vi "SCC Compare VIs.vi"(4 "version":string, 6 "interactive? (F)":bool, 7 "application reference":refnum<vi>, 8 "error in (no error)":errorcluster, 9 "compare options":T1={"VI Attributes"=FALSE, "Front Panel"=TRUE, "FP position/size"=FALSE, "Block Diagram"=TRUE, "BD cosmetic"=FALSE, "BD position/size"=FALSE}, 10 "VI path":path, 11 "source control reference in":T2) -> (0 "error out":errorcluster, 2 "status message":string, 3 "source control reference out":T2, 5 "file differs?":bool)   [LabVIEW 2017, in "NI_SCC.lvlib"]
doc: "Returns the difference between the specified VI and by default, the latest version of the VI in source control."
uses:
  <vilib>/SourceControl/sccapi/NI_SCC.lvlib
  <vilib>/SourceControl/sccapi/SCCAPI Refnum.ctl
  <vilib>/SourceControl/sccapi/SCCAPI VI Compare Options.ctl
  <vilib>/SourceControl/sccapi/SCCAPI SCC Provider Functionality.ctl
  <vilib>/SourceControl/support/SCCSup Message Strings GLBL.vi
  <vilib>/Utility/lvfile.llb/NI_FileType.lvlib
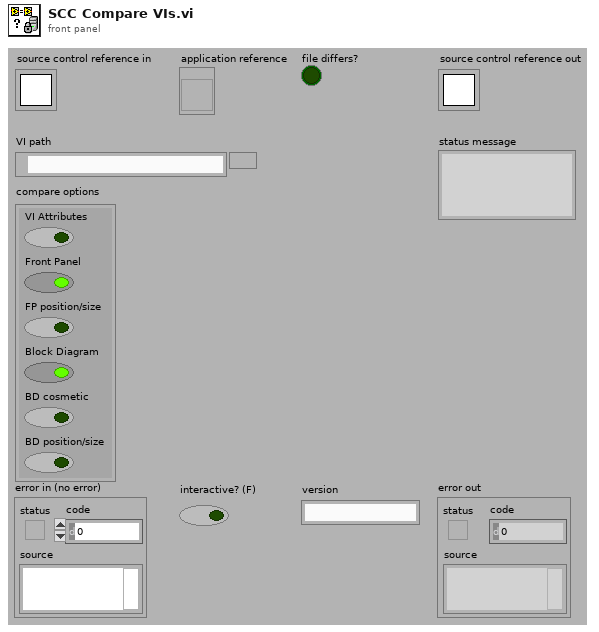
[diagram p1: front panel]
types:
  T1 = typedef "NI_SCC.lvlib/SCCAPI VI Compare Options.ctl" = cluster{"VI Attributes":bool, "Front Panel":bool, "FP position/size":bool, "Block Diagram":bool, "BD cosmetic":bool, "BD position/size":bool}
  T2 = typedef "NI_SCC.lvlib/SCCAPI Refnum.ctl" = refnum<k1>
  T3 = typedef "NI_SCC.lvlib/SCCAPI SCC Provider Functionality.ctl" = enum16{"Advanced - Get Latest", "Advanced - CheckOut", "Advanced - CheckIn", "Advanced - UndoCheckOut", "Advanced - Add", "Advanced - Remove", "Advanced - FileCompare", "Advanced - FileHistory", "Advanced - FileProperties", "Advanced - ConfigOptions", "Run SCC", "Configure Project", "Comment on CheckOut", "Comment on CheckIn", "Comment on Add", "Comment on Remove", "Keep Checked Out", "Get File Copy", "Multifile History"}
  T4 = typedef "NI_SCC.lvlib/SCCAPI SCC File Status.ctl" = cluster{"in source control?":bool, "checked out by user?":bool, "checked out by other?":bool, "out of date?":bool, "deleted?":bool}
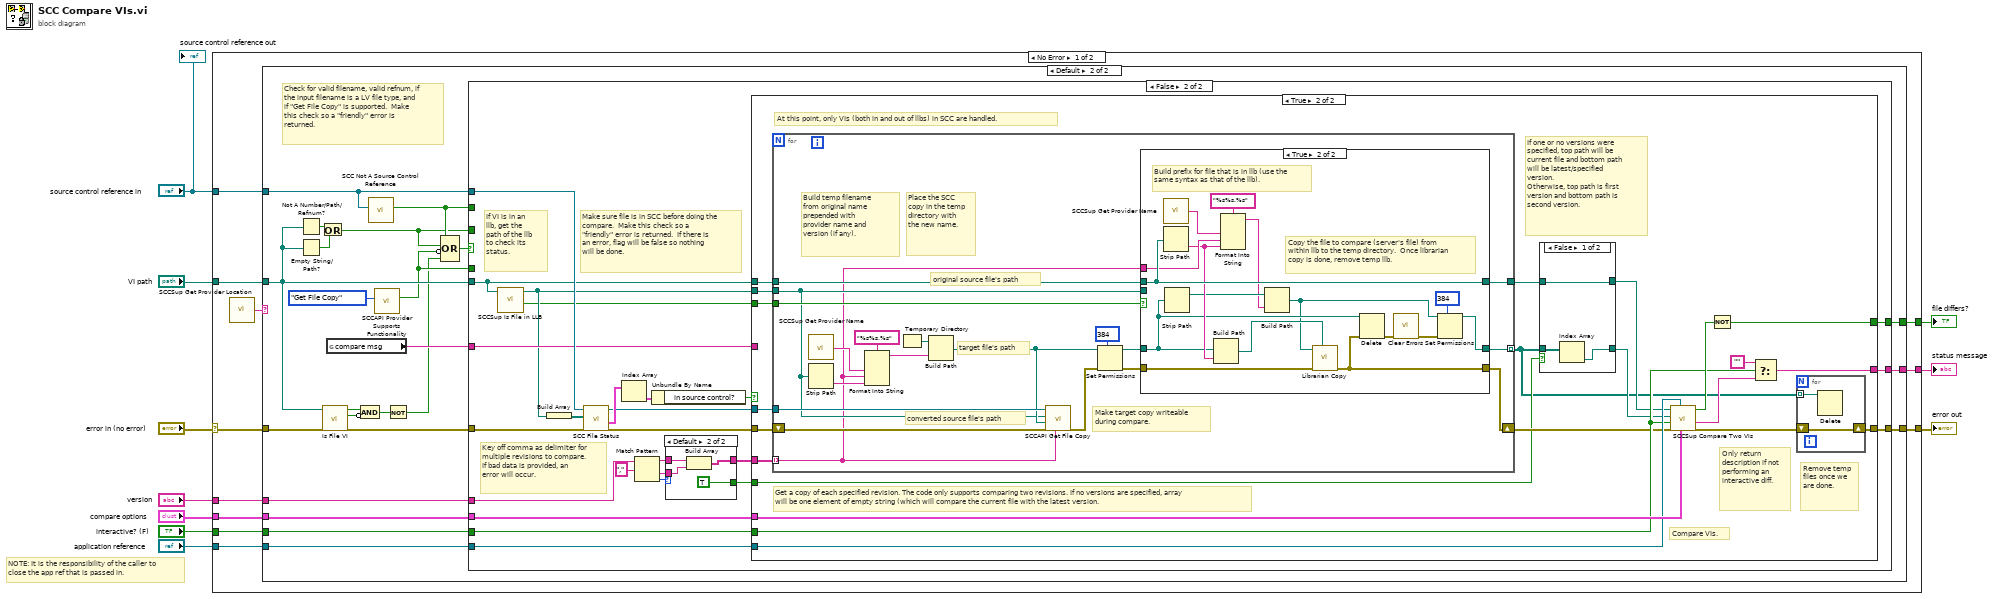
[diagram p0: block diagram]
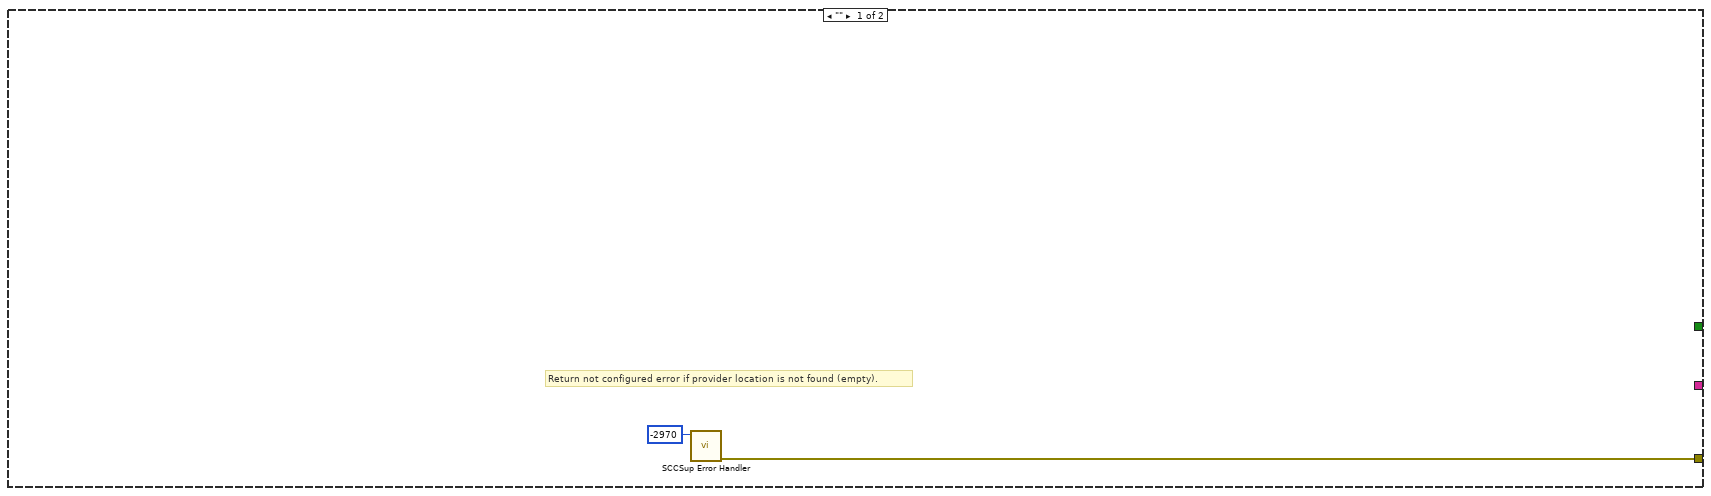
[diagram p2: hidden frame]
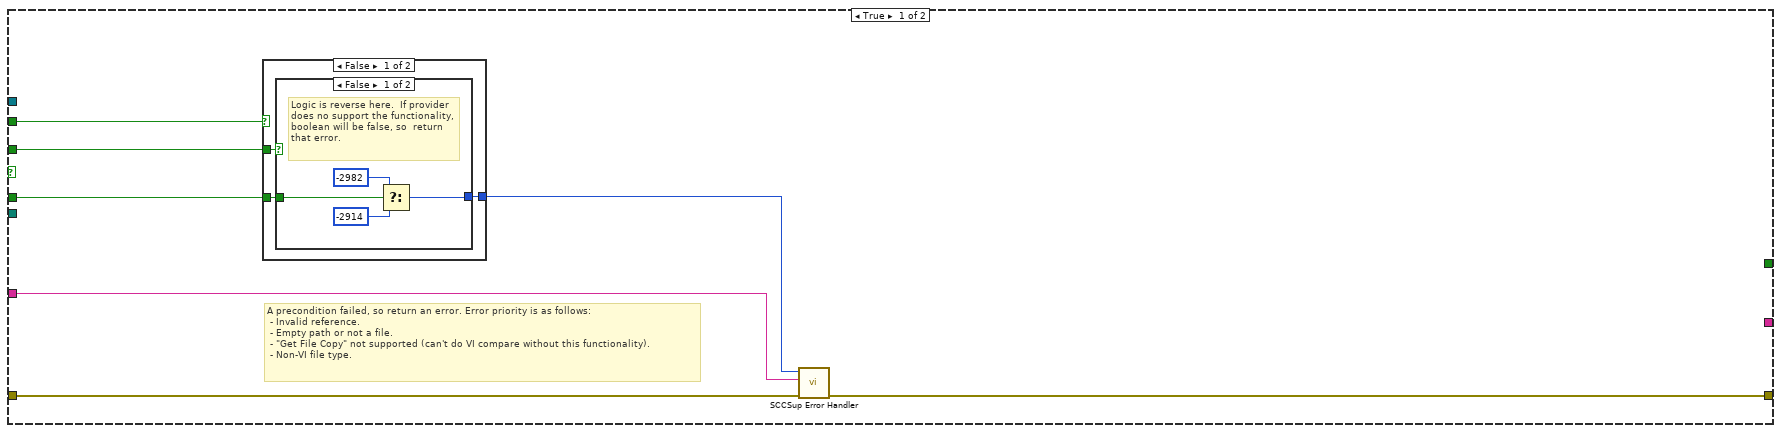
[diagram p3: hidden frame]
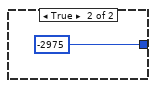
[diagram p4: hidden frame]
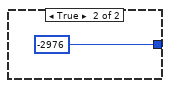
[diagram p5: hidden frame]
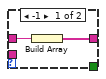
[diagram p6: hidden frame]
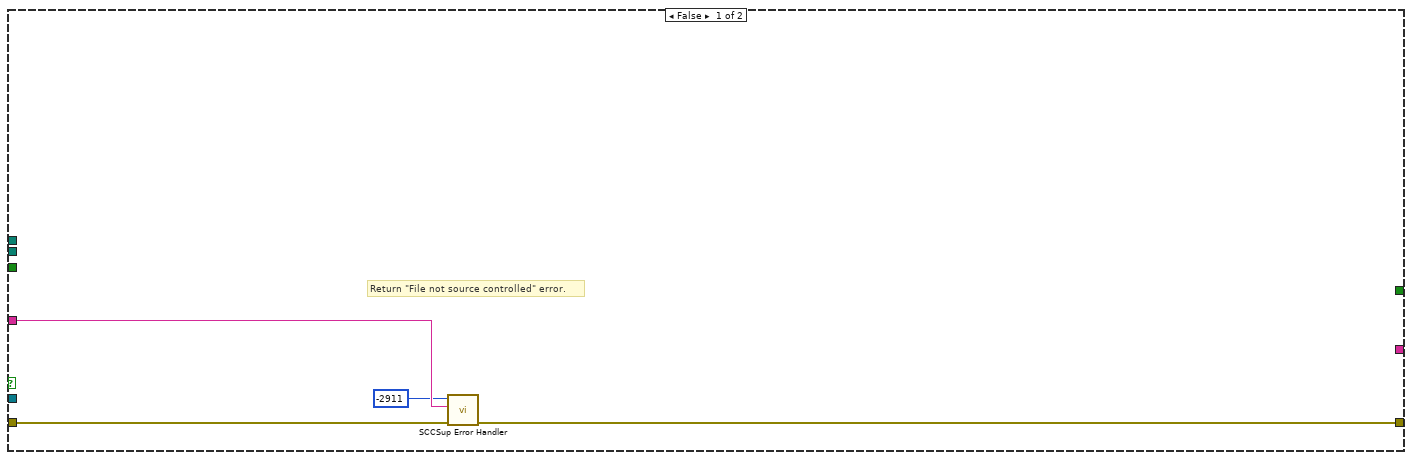
[diagram p7: hidden frame]
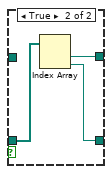
[diagram p8: hidden frame]
diagram:
  # "NOTE: It is the responsibility of the caller to close the app ref that is passed in."
  n1 = case shown="No Error" "error in (no error)" {
    selector: "error in (no error)" -> [w14 w166]
    tunnel: [w18 w166] -> w4
    tunnel: "source control reference in" -> [w21 _]
    tunnel: [w20 _] -> w3
    tunnel: "VI path" -> [w13 _]
    tunnel: [w19 _] -> w2
    tunnel: "compare options" -> [w16 _]
    tunnel: "interactive? (F)" -> [w17 _]
    tunnel: "version" -> [w15 _]
    tunnel: "application reference" -> [w12 _]
    frame No Error {
      n2 = call <vilib>:"SCCSup Get Provider Location.vi"() -> ("provider location"=w11:string)  [unwired: 6 in]
      n3 = case shown="Default" w11 {
        tunnel: w21 -> [_ w44]
        tunnel: [_ w41] -> w20
        tunnel: [_ w40] -> w19
        tunnel: [w22 w39] -> w18
        tunnel: w17 -> [_ w38]
        tunnel: w16 -> [_ w37]
        tunnel: w15 -> [_ w36]
        tunnel: w14 -> [_ w34]
        tunnel: w13 -> [_ w32]
        tunnel: w12 -> [_ w28]
        frame "" {
          # "Return not configured error if provider location is not found (empty)."
          n4 = call <vilib>:"SCCSup Error Handler.vi"("scc error code"=-2970 ("code")) -> ("error out"=w22:errorcluster)  [unwired: 10 in]
        }
        frame Default {
          # "Check for valid filename, valid refnum, if the input filename is a LV file type, and if \"Get File Copy\" is supported.  Make this check so a \"friendly\" error is returned."
          n5 = Not A Number/Path/Refnum?(number/path/refnum=w32) -> (NaN/Path/Refnum?=w46:bool)
          n6 = Empty String/Path?(string/path=w32) -> (empty?=w45:bool)
          n7 = Or(x=w46, y=w45) -> (x .or. y?=w31:bool)
          n8 = call <vilib>:"Is File VI.vi"("error in (no error)"=w34, "path"=w32) -> ("error out"=w33:errorcluster, "Is Class Private Data Control?"=w25:bool, "Is VI?"=w26:bool)  [unwired: 7 in]
          n9 = global read "SCCSup Message Strings GLBL.vi" "compare msg"() -> (w35:string)
          n10 = Compound Arithmetic op=AND(w26, invert w25) -> (w24:bool)
          n11 = call <vilib>:"SCC Not A Source Control Reference.vi"("source control reference in"=w44) -> ("not a source control reference?"=w42:bool)  [unwired: 9 in, 1 out]
          n12 = call <vilib>:"SCCAPI Provider Supports Functionality.vi"("functionality"=SCCAPI_SCC_Provider_Functionality."Get File Copy") -> ("provider supports?"=w29:bool)  [unwired: 9 in, 1 out]
          n13 = Not(x=w24) -> (.not. x?=w27:bool)
          n14 = Compound Arithmetic op=OR(w42, w31, invert w29, w27) -> (w43:bool)
          n15 = case shown="False" w43 {
            tunnel: w44 -> [_ w79]
            tunnel: [_ w80] -> w41
            tunnel: w32 -> [_ w72]
            tunnel: w42 -> [w50 _]
            tunnel: [_ w81] -> w40
            tunnel: w33 -> [w53 w76]
            tunnel: [w52 w82] -> w39
            tunnel: w38 -> [_ w87]
            tunnel: w37 -> [_ w86]
            tunnel: w36 -> [_ w68]
            tunnel: w35 -> [w51 w77]
            tunnel: w31 -> [w49 _]
            tunnel: w29 -> [w47 _]
            tunnel: w28 -> [_ w73]
            frame True {
              # "A precondition failed, so return an error. Error priority is as follows:\n - Invalid reference.  \n - Empty path or not a file.\n - \"Get File Copy\" not supported (can't do VI compare without this functionality).\n - Non-VI file type."
              n16 = case shown="False" w50 {
                tunnel: w49 -> [w54 _]
                tunnel: [w56 -2976 ("result")] -> w48
                tunnel: w47 -> [w55 _]
                frame False {
                  n17 = case shown="False" w54 {
                    tunnel: [w58 -2975 ("result")] -> w56
                    tunnel: w55 -> [w57 _]
                    frame False {
                      # "Logic is reverse here.  If provider does no support the functionality, boolean will be false, so  return that error."
                      n18 = Select(t=-2982 ("result"), s=w57, f=-2914 ("result")) -> (s? t:f=w58:i32)
                    }
                    frame True {
                    }
                  }
                }
                frame True {
                }
              }
              n19 = call <vilib>:"SCCSup Error Handler.vi"("error in (no error)"=w53, "operation message"=w51, "scc error code"=w48) -> ("error out"=w52:errorcluster)  [unwired: 8 in]
            }
            frame False {
              # "Key off comma as delimiter for multiple revisions to compare. If bad data is provided, an error will occur."
              # "If VI is in an llb, get the path of the llb to check its status."
              # "Make sure file is in SCC before doing the compare.  Make this check so a \"friendly\" error is returned.  If there is an error, flag will be false so nothing will be done."
              n20 = call <vilib>:"SCCSup Is File in LLB.vi"("Path"=w72) -> ("is in LLB?"=w70:bool, "converted path"=w71:path)  [unwired: 9 in]
              n21 = Build Array(w71) -> (w85:path[])
              n22 = call <vilib>:"SCC File Status.vi"("error in (no error)"=w76, "files"=w85, "source control reference in"=w79) -> ("error out"=w74:errorcluster, "file status"=w83:T4[], "source control reference out"=w78:T2)  [unwired: 4 in, 2 out]
              n23 = Index Array(array=w83) -> (element=w84:T4)  [unwired: 1 in]
              n24 = Match Pattern(string=w68, regular expression=",") -> (before substring=w66:string, after substring=w65:string, offset past match=w67:i32)  [unwired: 1 in, 1 out]
              n25 = Unbundle By Name(w84) -> ("in source control?"=w75:bool)
              n26 = case shown="Default" w67 {
                tunnel: w66 -> [w89 w93]
                tunnel: w65 -> [_ w92]
                tunnel: [w88 w91] -> w64
                tunnel: [_ TRUE] -> w63
                frame -1 {
                  n27 = Build Array(w89) -> (w88:string[])
                }
                frame Default {
                  n28 = Build Array(w93, w92) -> (w91:string[])
                }
              }
              n29 = case shown="True" w75 {
                tunnel: w87 -> [_ w107]
                tunnel: w86 -> [_ w117]
                tunnel: w74 -> [w97 w118]
                tunnel: [w96 w99] -> w82
                tunnel: w77 -> [w95 _]
                tunnel: [_ w115] -> w81
                tunnel: [_ w112] -> w80
                tunnel: w78 -> [_ w119]
                tunnel: w72 -> [_ w108]
                tunnel: w73 -> [_ w111]
                tunnel: w71 -> [_ w109]
                tunnel: w70 -> [_ w110]
                tunnel: w64 -> [_ w105]
                tunnel: w63 -> [_ w104]
                frame False {
                  # "Return \"File not source controlled\" error."
                  n30 = call <vilib>:"SCCSup Error Handler.vi"("error in (no error)"=w97, "operation message"=w95, "scc error code"=-2911 ("error code")) -> ("error out"=w96:errorcluster)  [unwired: 8 in]
                }
                frame True {
                  # "If one or no versions were specified, top path will be current file and bottom path will be latest/specified version.\nOtherwise, top path is first version and bottom path is second version."
                  # "Get a copy of each specified revision. The code only supports comparing two revisions. If no versions are specified, array will be one element of empty string (which will compare the current file with the latest version."
                  # "Compare VIs."
                  # "Only return description if not performing an interactive diff."
                  # "Remove temp files once we are done."
                  # "At this point, only VIs (both in and out of llbs) in SCC are handled."
                  n31 = for {
                    tunnel: w119 -> [w146]
                    tunnel: w110 -> [w136]
                    tunnel: w109 -> [w135]
                    tunnel: [w133] -> w103
                    tunnel: [w132] -> w98 mode=indexing
                    tunnel: w108 -> [w131]
                    shift-right: [w129] -> w106
                    shift-left: w118 -> [w144]
                    tunnel: w105 -> [w128] mode=indexing
                    # "original source file's path"
                    # "Make target copy writeable during compare."
                    # "target file's path"
                    # "Build temp filename from original name prepended with provider name and version (if any)."
                    # "converted source file's path"
                    # "Place the SCC copy in the temp directory with the new name."
                    n32 = call <vilib>:"SCCSup Get Provider Name.vi"() -> ("provider name"=w137:string)  [unwired: 6 in]
                    n33 = Strip Path(path=w135) -> (name=w139:string)  [unwired: 1 out]
                    n34 = Format Into String(format string="%s%s.%s", w137, w128, w139) -> (resulting string=w138:string)  [unwired: 2 in, 1 out]
                    n35 = Temporary Directory() -> (w145:path)
                    n36 = Build Path(base path=w145, name or relative path=w138) -> (appended path=w141:path)
                    n37 = call <vilib>:"SCCAPI Get File Copy.vi"("version"=w128, "error in (no error)"=w144, "target filename"=w141, "source filename"=w135, "source control reference in"=w146) -> ("error out"=w142:errorcluster)  [unwired: 4 in, 2 out]
                    n38 = Set Permissions(7:i16 384 ("x"), 8:w142, 11:w141) -> (0:w130:errorcluster, 3:w134:path)  [unwired: 2 in]
                    n39 = case shown="True" w136 {
                      tunnel: w135 -> [w149 _]
                      tunnel: w134 -> [w148 w156]
                      tunnel: [w149 w163] -> w133
                      tunnel: [w148 w153] -> w132
                      tunnel: w131 -> [_ w163]
                      tunnel: w128 -> [_ w162]
                      tunnel: w130 -> [w147 w157]
                      tunnel: [w147 w152] -> w129
                      frame False {
                        # "target file's path"
                        # "converted source file's path"
                      }
                      frame True {
                        # "Copy the file to compare (server's file) from within llb to the temp directory.  Once librarian copy is done, remove temp llb."
                        # "Build prefix for file that is in llb (use the same syntax as that of the llb)."
                        n40 = call <vilib>:"SCCSup Get Provider Name.vi"() -> ("provider name"=w165:string)  [unwired: 6 in]
                        n41 = Strip Path(path=w163) -> (name=w161:string)  [unwired: 1 out]
                        n42 = Strip Path(path=w156) -> (stripped path=w160:path)  [unwired: 1 out]
                        n43 = Build Path(base path=w156, name or relative path=w161) -> (appended path=w158:path)
                        n44 = Format Into String(format string="%s%s.%s", w165, w162, w161) -> (resulting string=w159:string)  [unwired: 2 in, 1 out]
                        n45 = Build Path(base path=w160, name or relative path=w159) -> (appended path=w154:path)
                        n46 = call <vilib>:"Librarian Copy.vi"("source"=w158, "error in (no error)"=w157, "destination"=w154) -> ("error out"=w152:errorcluster)  [unwired: 7 in, 1 out]
                        n47 = Delete(path (use dialog)=w156, error in=w152) -> (error out=w151:errorcluster)  [unwired: 3 in, 2 out]
                        n48 = call <vilib>:"Clear Errors.vi"("error in (no error)"=w151) -> ("error out"=w150:errorcluster)  [unwired: 5 in, 1 out]
                        n49 = Set Permissions(7:i16 384 ("x"), 8:w150, 11:w154) -> (3:w153:path)  [unwired: 2 in, 1 out]
                      }
                    }
                  }
                  n50 = case shown="False" w104 {
                    tunnel: w98 -> [w123 w127]
                    tunnel: w103 -> [w124 _]
                    tunnel: [w124 w126] -> w102
                    tunnel: [w122 w125] -> w101
                    frame False {
                      n51 = Index Array(array=w123) -> (element=w122:path)  [unwired: 1 in]
                    }
                    frame True {
                      n52 = Index Array(array=w127) -> (element #1=w126:path, element #2=w125:path)  [unwired: 2 in]
                    }
                  }
                  n53 = call <vilib>:"SCCSup Compare Two VIs.vi"("compare options"=w117, "application reference"=w111, "error in (no error)"=w106, "Interactive (F)"=w107, "Second VI"=w101, "First VI"=w102) -> ("error out"=w100:errorcluster, "description"=w114:string, "Same?"=w116:bool)  [unwired: 3 in]
                  n54 = Not(x=w116) -> (.not. x?=w115:bool)
                  n55 = Select(t="", s=w107, f=w114) -> (s? t:f=w112:string)
                  n56 = for {
                    shift-right: [w121] -> w99
                    shift-left: w100 -> [w121]
                    tunnel: w98 -> [w120] mode=indexing
                    n57 = Delete(path (use dialog)=w120) -> ()  [unwired: 4 in, 3 out]
                  }
                }
              }
            }
          }
        }
      }
    }
    frame Error {
    }
  }
  "error out" <- w4
  "status message" <- w3
  "file differs?" <- w2
  "source control reference out" <- "source control reference in"
